vi "IBM4_Read(V1).vi"(8 "error in":errorcluster, 10 "Channel":i32, 11 "COM resource in":refnum<visa-resource-name>="COM9") -> (0 "error out":errorcluster, 2 "output":dbl, 3 "COM resource out":refnum<visa-resource-name>)   [LabVIEW 2022 SP3, in "IBM4.lvlib"]
doc: "This VI interfaces with the IBM4 to perform a read operation.\n\nThe input channel must be between 0 and 3, while the output will in floating point format (thus, in Voltss).\nOnly a single read operation is made with this VI. \n\nAlternate read operations exist covering binary or floating point, single reading, multiple readings, and an average of multiple readings (floating point only)."
uses:
  <instrlib>/IBM4/IBM4.lvlib
panel:
  out "error out 2":errorcluster
  out "read buffer":string
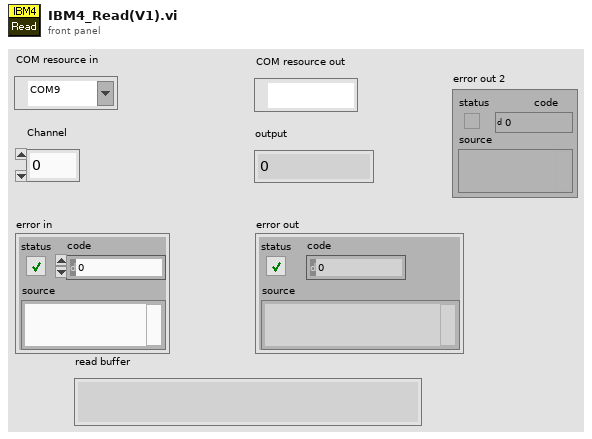
[diagram p1: front panel]
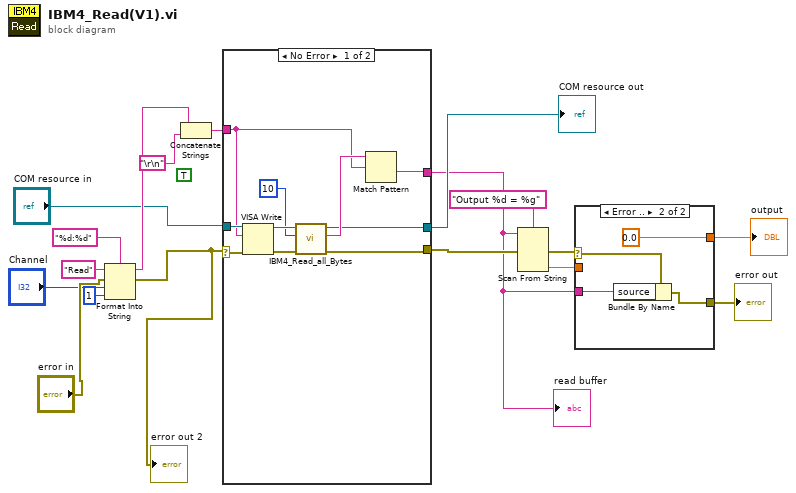
[diagram p0: block diagram]
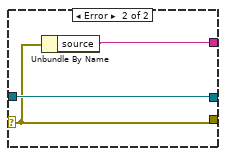
[diagram p3: hidden frame]
diagram:
  (unwired) TRUE ("Enable Termination\nChar (T)")
  n1 = Format Into String(format string="%d:%d", initial string="Read", error in="error in", "Channel", 1 ("input 2")) -> (resulting string=w9:string, error out=w1:errorcluster)
  "error out 2" <- w1
  n2 = Concatenate Strings(w9, "\r\n") -> (w8:string)
  n3 = case shown="No Error" w1 {
    selector: w1 -> [w23 w29]
    tunnel: "COM resource in" -> [w24 w31]
    tunnel: [w21 w29] -> w12
    tunnel: [w19 w30] -> w3
    tunnel: w8 -> [w22 _]
    tunnel: [w20 w31] -> w13
    frame No Error {
      n4 = VISA Write(VISA resource name=w24, write buffer=w22, error in (no error)=w23) -> (VISA resource name out=w27:refnum<visa-resource-name>, error out=w28:errorcluster)  [unwired: 1 out]
      n5 = call <instrlib>:"IBM4_Read_all_Bytes.vi"("error in (no error)"=w28, "milliseconds to wait"=u32 10, "VISA Refnum in"=w27) -> ("error out"=w21:errorcluster, "String"=w26:string, "VISA Refnum out"=w20:refnum<visa-resource-name>)  [unwired: 2 in]
      n6 = Match Pattern(string=w26, regular expression=w22) -> (after substring=w19:string)  [unwired: 1 in, 3 out]
    }
    frame Error {
      n7 = Unbundle By Name(w29) -> ("source"=w30:string)
    }
  }
  "COM resource out" <- w13
  "read buffer" <- w3
  n8 = Scan From String(format string="Output %d = %g", input string=w3, error in=w12) -> (error out=w7:errorcluster, output 2=w6:dbl)  [unwired: 4 in, 2 out]
  n9 = case shown="Error .." w7 {
    selector: w7 -> [w32 w36]
    tunnel: w6 -> [w33 _]
    tunnel: [w33 0.0] -> w5
    tunnel: [w32 w34] -> w4
    tunnel: w3 -> [_ w35]
    frame No Error {
    }
    frame Error {
      n10 = Bundle By Name(cluster=w36, "source"=w35) -> (w34:errorcluster)
    }
  }
  "error out" <- w4
  "output" <- w5
